vi "Main.vi"() -> ()   [LabVIEW 2016]
uses:
  Data Highway TD.ctl
  Queue Attributes TD.ctl
  Que Enum td.ctl
panel:
  in  "Log":bool
  in  "PP_value":dbl
  in  "PP_HOME":bool
  in  "PP_STOP":bool
  in  "PP_START":bool
  in  "Connect":bool
  in  "Exit":bool
  # "Pitchpack"
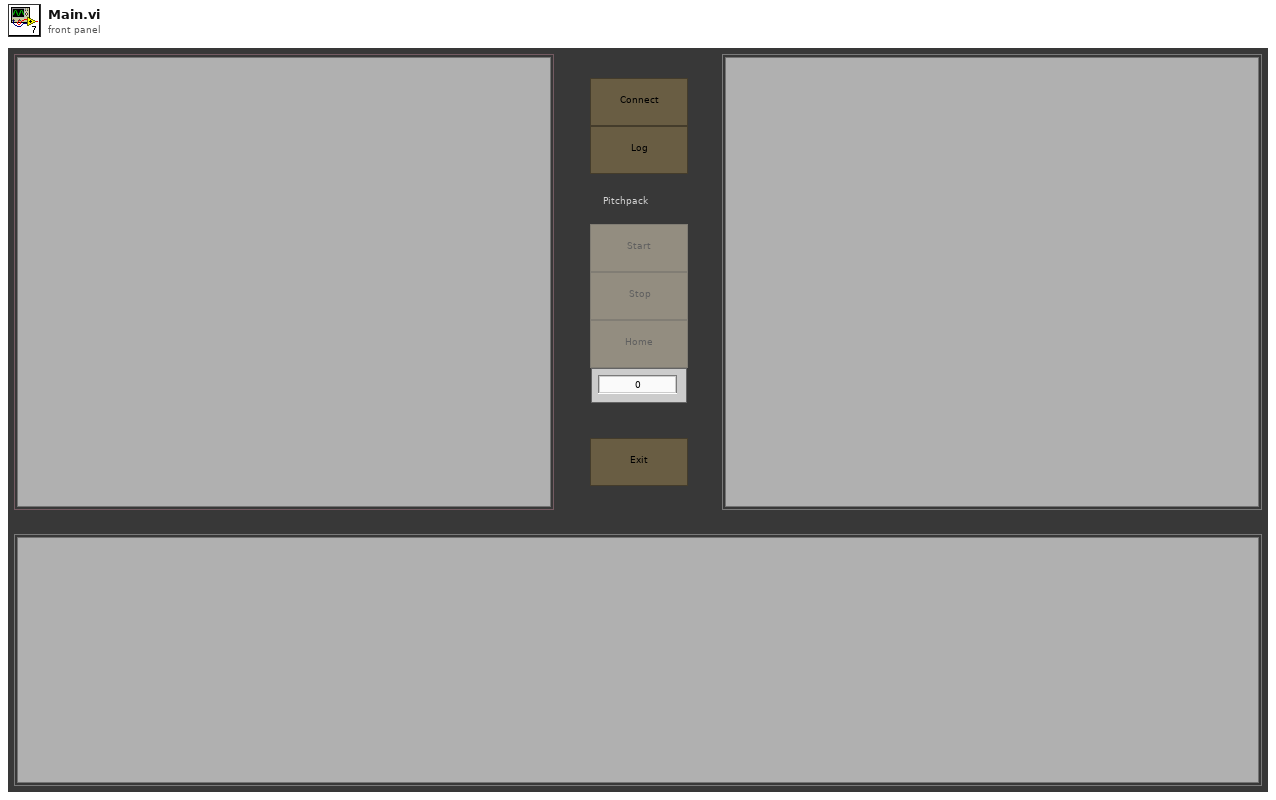
[diagram p1: front panel]
types:
  T1 = typedef "Data Highway TD.ctl" = cluster{"PP_value":dbl, "String":string, "Boolean":bool}
  T2 = typedef "Que Cluster TD.ctl" = cluster{"Main":refnum<queue>, "ZMQ_SUB":refnum<queue>, "External":refnum<queue>, "Vibration":refnum<queue>, "ZMQ_REQ":refnum<queue>}
  T3 = typedef "Queue Attributes TD.ctl" = cluster{"Que States":T4, "String":string, "Boolean":bool, "Double":dbl, "U16":u16}
  T4 = typedef "Que enum td.ctl" = enum16{"Stop", "Start", "Update D_HW", "Initialize", "Exit", "Read", "Write", "Plot", "Log", "Stop Log", "Start Log", "Wait"}
  T5 = typedef "Que Atributes TD.ctl" = cluster{"Que States":T4, "String":string, "Boolean":bool, "Double":dbl, "U16":u16}
  T6 = enum8{"Enabled", "Disabled", "Disabled and Grayed Out"}
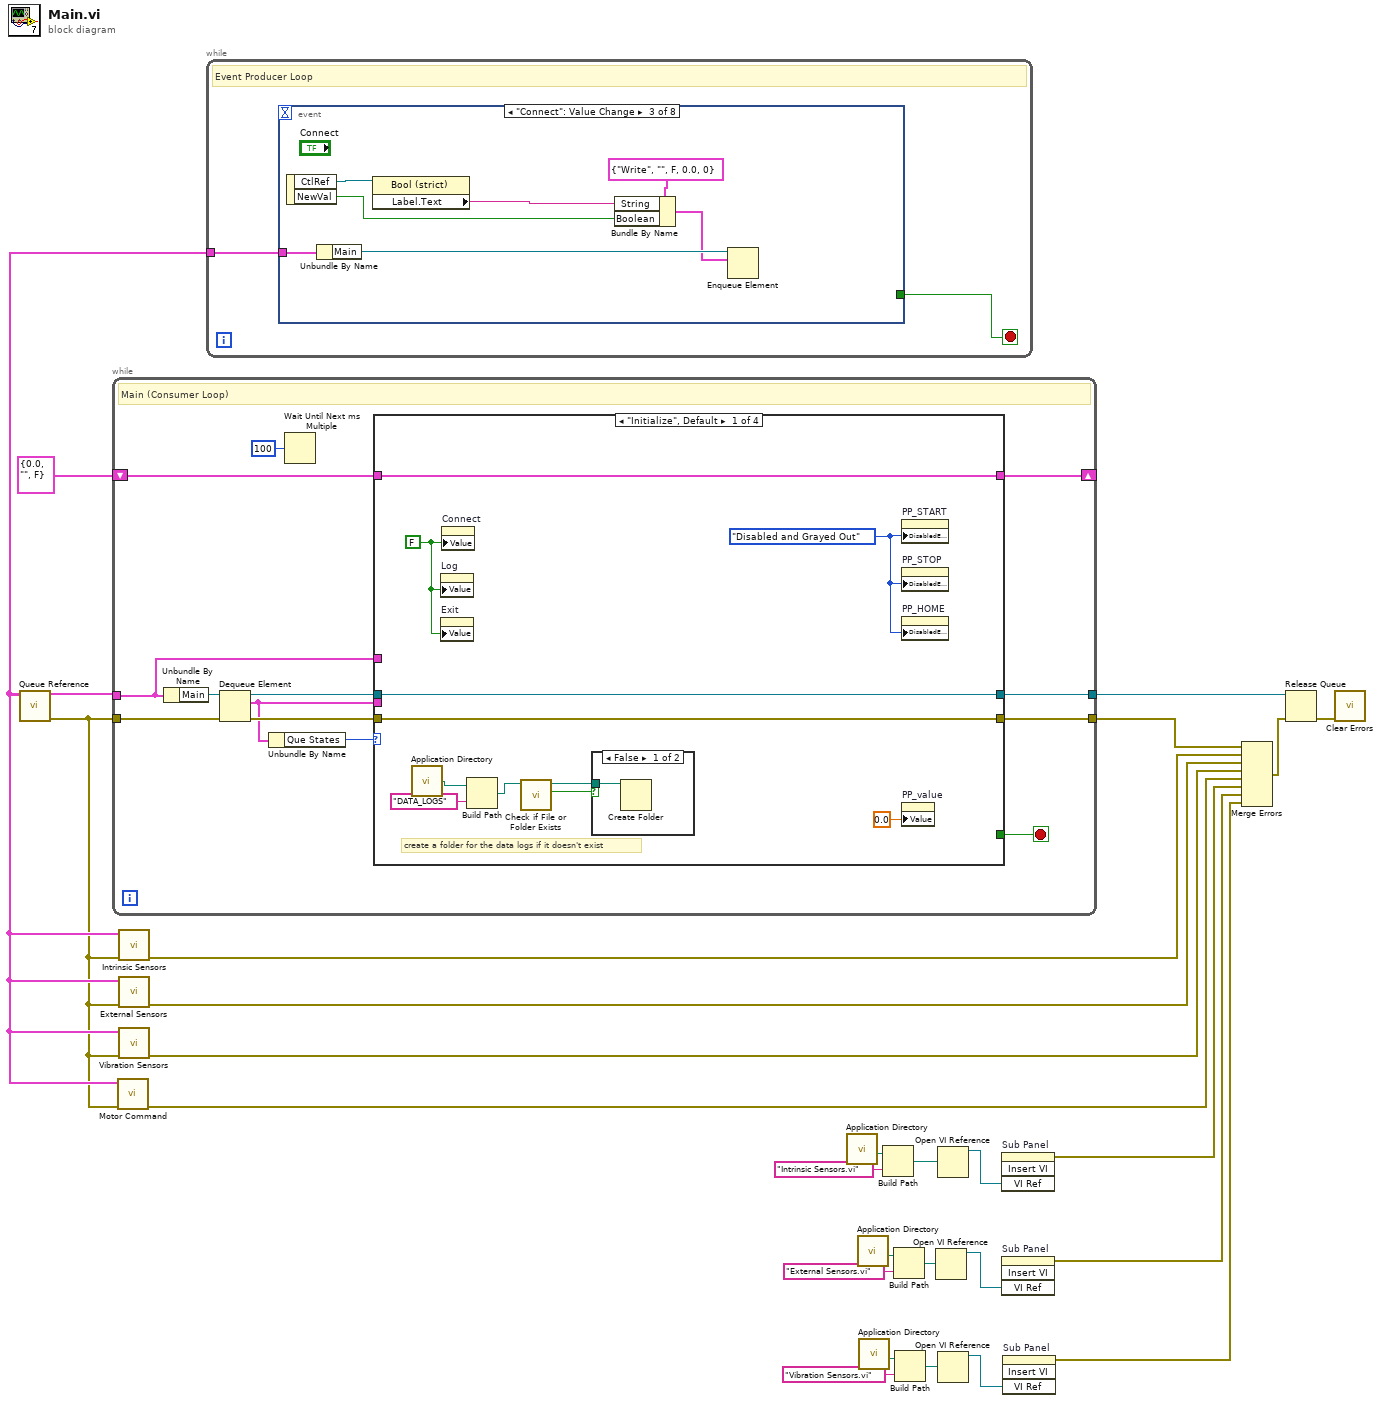
[diagram p0: block diagram]
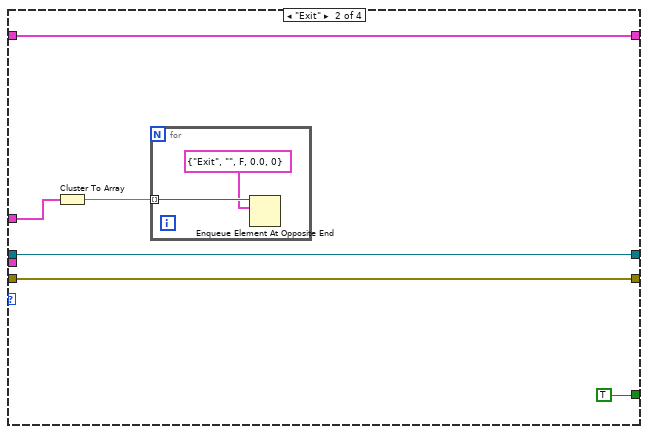
[diagram p3: hidden frame]
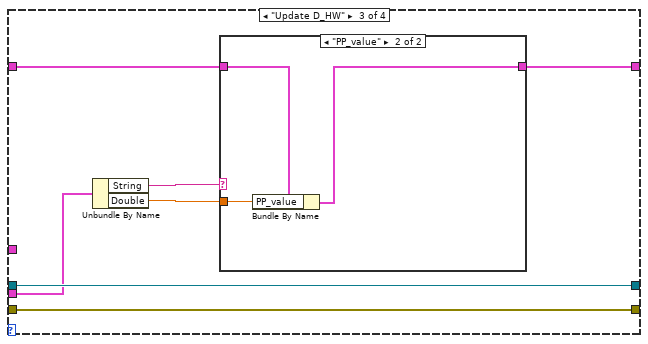
[diagram p4: hidden frame]
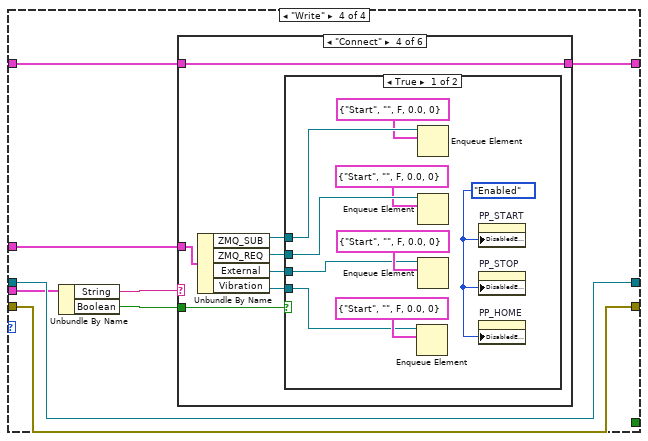
[diagram p6: hidden frame]
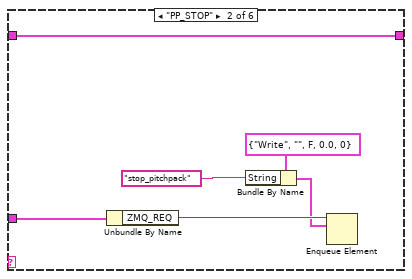
[diagram p8: hidden frame]
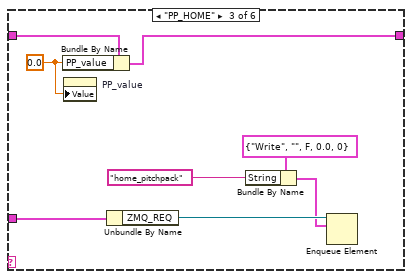
[diagram p9: hidden frame]
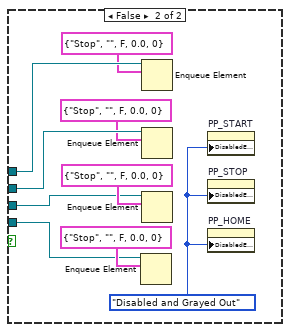
[diagram p10: hidden frame]
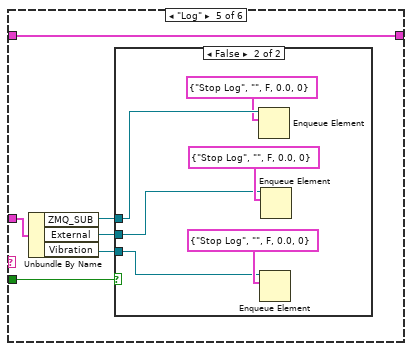
[diagram p11: hidden frame]
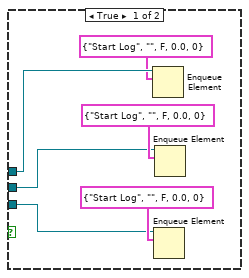
[diagram p12: hidden frame]
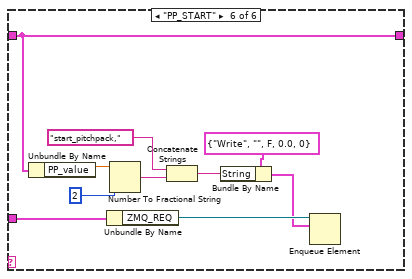
[diagram p13: hidden frame]
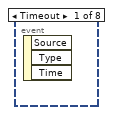
[diagram p14: hidden frame]
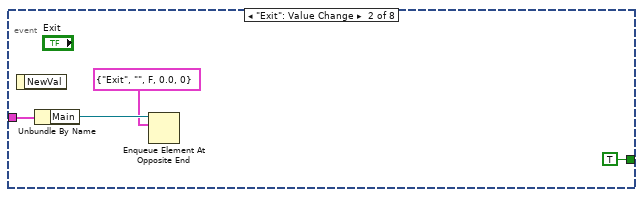
[diagram p15: hidden frame]
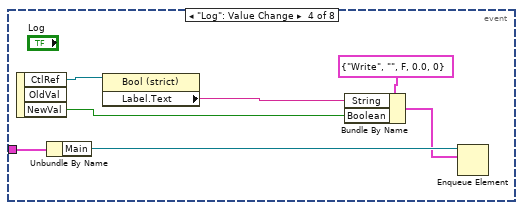
[diagram p16: hidden frame]
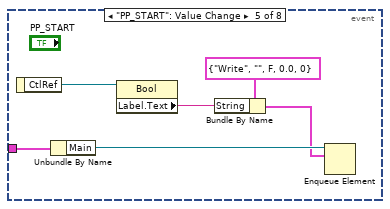
[diagram p17: hidden frame]
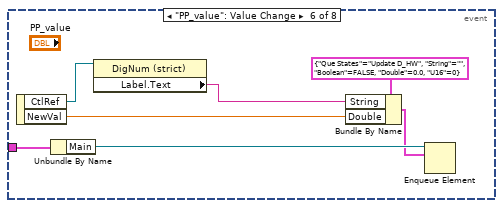
[diagram p18: hidden frame]
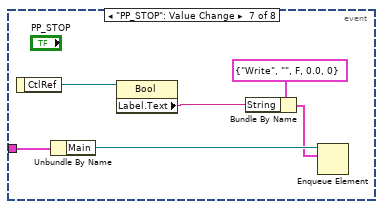
[diagram p19: hidden frame]
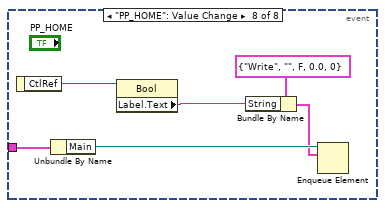
[diagram p20: hidden frame]
diagram:
  n1 = call "Queue Reference.vi"() -> ("error out"=w2:errorcluster, "output cluster"=w3:T2)  [unwired: 10 in]
  n2 = while {
    tunnel: w2 -> [w38]
    tunnel: w3 -> [w32]
    tunnel: [w35] -> w26
    tunnel: [w34] -> w24
    shift-right: [w30] -> _
    shift-left: T1 {"PP_value"=0.0, "String"="", "Boolean"=FALSE} ("Data Hyway") -> [w31]
    stop <- w28 stop-if-true
    # "Main (Consumer Loop)"
    n3 = Unbundle By Name(w32) -> ("Main"=w39:refnum<queue>)
    n4 = Dequeue Element(queue=w39, error in (no error)=w38) -> (queue out=w37:refnum<queue>, element=w27:T5, error out=w36:errorcluster)  [unwired: 1 in, 1 out]
    n5 = Unbundle By Name(w27) -> ("Que States"=w33:T4)
    n6 = Wait Until Next ms Multiple(millisecond multiple=u32 100) -> ()  [unwired: 1 out]
    n7 = case shown="\"Initialize\", Default" w33 {
      tunnel: w37 -> [w50 w57 w66 w77]
      tunnel: w36 -> [w49 w56 w63 w72]
      tunnel: [w50 w57 w66 w77] -> w35
      tunnel: [w49 w56 w63 w72] -> w34
      tunnel: w32 -> [_ w54 _ w78]
      tunnel: w31 -> [w48 w55 w65 w76]
      tunnel: [w48 w55 w64 w75] -> w30
      tunnel: [_ TRUE _ _] -> w28
      tunnel: w27 -> [_ _ w62 w74]
      frame "Initialize", Default {
        w45 = FALSE ("Connect")
        w47 = T6."Disabled and Grayed Out" ("Disabled")
        # "create a folder for the data logs if it doesn't exist"
        n8 = call <vilib>:"Application Directory.vi"() -> ("Application Directory"=w42:path)
        n9 = property on="Log" class="Bool (strict)"("Value"=w45) -> ()  [unwired: 2 in, 2 out]
        n10 = property on="Exit" class="Bool (strict)"("Value"=w45) -> ()  [unwired: 2 in, 2 out]
        n11 = property on="Connect" class="Bool (strict)"("Value"=w45) -> ()  [unwired: 2 in, 2 out]
        n12 = Build Path(base path=w42, name or relative path="DATA_LOGS") -> (appended path=w44:path)
        n13 = call <vilib>:"Check if File or Folder Exists.vi"("path"=w44) -> ("file or folder exists?"=w41:bool, "dup path"=w40:path)  [unwired: 8 in, 1 out]
        n14 = case shown="False" w41 {
          tunnel: w40 -> [w51 _]
          frame False {
            n15 = Create Folder(path (use dialog)=w51) -> ()  [unwired: 2 in, 3 out]
          }
          frame True {
          }
        }
        n16 = property on="PP_START" class="Bool"("DisabledEnum"=w47) -> ()  [unwired: 2 in, 2 out]
        n17 = property on="PP_STOP" class="Bool"("DisabledEnum"=w47) -> ()  [unwired: 2 in, 2 out]
        n18 = property on="PP_HOME" class="Bool"("DisabledEnum"=w47) -> ()  [unwired: 2 in, 2 out]
        n19 = property on="PP_value" class="DigNum (strict)"("Value"=0.0 ("PP_value")) -> ()  [unwired: 2 in, 2 out]
      }
      frame "Exit" {
        n20 = Cluster To Array(cluster=w54) -> (array=w53:refnum<queue>[])
        n21 = for {
          tunnel: w53 -> [w59] mode=indexing
          n22 = Enqueue Element At Opposite End(queue=w59, element=T3 {"Que States"=enum."Exit", "String"="", "Boolean"=FALSE, "Double"=0.0, "U16"=0}) -> ()  [unwired: 2 in, 3 out]
        }
      }
      frame "Update D_HW" {
        n23 = Unbundle By Name(w62) -> ("String"=w61:string, "Double"=w60:dbl)
        n24 = case shown="\"PP_value\"" w61 {
          tunnel: w65 -> [w67 w70]
          tunnel: [w67 w69] -> w64
          tunnel: w60 -> [_ w68]
          frame "False", Default {
          }
          frame "PP_value" {
            n25 = Bundle By Name(cluster=w70, "PP_value"=w68) -> (w69:T1)
          }
        }
      }
      frame "Write" {
        n26 = Unbundle By Name(w74) -> ("String"=w73:string, "Boolean"=w71:bool)
        n27 = case shown="\"Connect\"" w73 {
          tunnel: w78 -> [_ w85 w93 w99 w123 w146]
          tunnel: w76 -> [w79 w82 w90 w100 w124 w141]
          tunnel: [w79 w82 w89 w100 w124 w141] -> w75
          tunnel: w71 -> [_ _ _ w96 w121 _]
          frame "False", Default {
          }
          frame "PP_STOP" {
            n28 = Unbundle By Name(w85) -> ("ZMQ_REQ"=w84:refnum<queue>)
            n29 = Bundle By Name(cluster=T3 {"Que States"=enum."Write", "String"="", "Boolean"=FALSE, "Double"=0.0, "U16"=0} ("element"), "String"="stop_pitchpack") -> (w80:T3)
            n30 = Enqueue Element(queue=w84, element=w80) -> ()  [unwired: 2 in, 3 out]
          }
          frame "PP_HOME" {
            w86 = 0.0 ("PP_value")
            n31 = Bundle By Name(cluster=w90, "PP_value"=w86) -> (w89:T1)
            n32 = property on="PP_value" class="DigNum (strict)"("Value"=w86) -> ()  [unwired: 2 in, 2 out]
            n33 = Unbundle By Name(w93) -> ("ZMQ_REQ"=w92:refnum<queue>)
            n34 = Bundle By Name(cluster=T3 {"Que States"=enum."Write", "String"="", "Boolean"=FALSE, "Double"=0.0, "U16"=0} ("element"), "String"="home_pitchpack") -> (w87:T3)
            n35 = Enqueue Element(queue=w92, element=w87) -> ()  [unwired: 2 in, 3 out]
          }
          frame "Connect" {
            n36 = Unbundle By Name(w99) -> ("ZMQ_SUB"=w98:refnum<queue>, "ZMQ_REQ"=w97:refnum<queue>, "External"=w95:refnum<queue>, "Vibration"=w94:refnum<queue>)
            n37 = case shown="True" w96 {
              tunnel: w98 -> [w109 w118]
              tunnel: w97 -> [w108 w117]
              tunnel: w95 -> [w103 w112]
              tunnel: w94 -> [w101 w110]
              frame True {
                w107 = T6."Enabled" ("Disabled")
                n38 = Enqueue Element(queue=w101, element=T3 {"Que States"=enum."Start", "String"="", "Boolean"=FALSE, "Double"=0.0, "U16"=0}) -> ()  [unwired: 2 in, 3 out]
                n39 = Enqueue Element(queue=w109, element=T3 {"Que States"=enum."Start", "String"="", "Boolean"=FALSE, "Double"=0.0, "U16"=0}) -> ()  [unwired: 2 in, 3 out]
                n40 = Enqueue Element(queue=w108, element=T3 {"Que States"=enum."Start", "String"="", "Boolean"=FALSE, "Double"=0.0, "U16"=0}) -> ()  [unwired: 2 in, 3 out]
                n41 = Enqueue Element(queue=w103, element=T3 {"Que States"=enum."Start", "String"="", "Boolean"=FALSE, "Double"=0.0, "U16"=0}) -> ()  [unwired: 2 in, 3 out]
                n42 = property on="PP_START" class="Bool"("DisabledEnum"=w107) -> ()  [unwired: 2 in, 2 out]
                n43 = property on="PP_STOP" class="Bool"("DisabledEnum"=w107) -> ()  [unwired: 2 in, 2 out]
                n44 = property on="PP_HOME" class="Bool"("DisabledEnum"=w107) -> ()  [unwired: 2 in, 2 out]
              }
              frame False {
                w116 = T6."Disabled and Grayed Out" ("Disabled")
                n45 = Enqueue Element(queue=w110, element=T3 {"Que States"=enum."Stop", "String"="", "Boolean"=FALSE, "Double"=0.0, "U16"=0}) -> ()  [unwired: 2 in, 3 out]
                n46 = Enqueue Element(queue=w118, element=T3 {"Que States"=enum."Stop", "String"="", "Boolean"=FALSE, "Double"=0.0, "U16"=0}) -> ()  [unwired: 2 in, 3 out]
                n47 = Enqueue Element(queue=w117, element=T3 {"Que States"=enum."Stop", "String"="", "Boolean"=FALSE, "Double"=0.0, "U16"=0}) -> ()  [unwired: 2 in, 3 out]
                n48 = Enqueue Element(queue=w112, element=T3 {"Que States"=enum."Stop", "String"="", "Boolean"=FALSE, "Double"=0.0, "U16"=0}) -> ()  [unwired: 2 in, 3 out]
                n49 = property on="PP_START" class="Bool"("DisabledEnum"=w116) -> ()  [unwired: 2 in, 2 out]
                n50 = property on="PP_STOP" class="Bool"("DisabledEnum"=w116) -> ()  [unwired: 2 in, 2 out]
                n51 = property on="PP_HOME" class="Bool"("DisabledEnum"=w116) -> ()  [unwired: 2 in, 2 out]
              }
            }
          }
          frame "Log" {
            n52 = Unbundle By Name(w123) -> ("ZMQ_SUB"=w122:refnum<queue>, "External"=w120:refnum<queue>, "Vibration"=w119:refnum<queue>)
            n53 = case shown="False" w121 {
              tunnel: w122 -> [w130 w136]
              tunnel: w120 -> [w127 w133]
              tunnel: w119 -> [w125 w131]
              frame True {
                n54 = Enqueue Element(queue=w130, element=T3 {"Que States"=enum."Start Log", "String"="", "Boolean"=FALSE, "Double"=0.0, "U16"=0}) -> ()  [unwired: 2 in, 3 out]
                n55 = Enqueue Element(queue=w125, element=T3 {"Que States"=enum."Start Log", "String"="", "Boolean"=FALSE, "Double"=0.0, "U16"=0}) -> ()  [unwired: 2 in, 3 out]
                n56 = Enqueue Element(queue=w127, element=T3 {"Que States"=enum."Start Log", "String"="", "Boolean"=FALSE, "Double"=0.0, "U16"=0}) -> ()  [unwired: 2 in, 3 out]
              }
              frame False {
                n57 = Enqueue Element(queue=w136, element=T3 {"Que States"=enum."Stop Log", "String"="", "Boolean"=FALSE, "Double"=0.0, "U16"=0}) -> ()  [unwired: 2 in, 3 out]
                n58 = Enqueue Element(queue=w131, element=T3 {"Que States"=enum."Stop Log", "String"="", "Boolean"=FALSE, "Double"=0.0, "U16"=0}) -> ()  [unwired: 2 in, 3 out]
                n59 = Enqueue Element(queue=w133, element=T3 {"Que States"=enum."Stop Log", "String"="", "Boolean"=FALSE, "Double"=0.0, "U16"=0}) -> ()  [unwired: 2 in, 3 out]
              }
            }
          }
          frame "PP_START" {
            n60 = Unbundle By Name(w141) -> ("PP_value"=w144:dbl)
            n61 = Unbundle By Name(w146) -> ("ZMQ_REQ"=w145:refnum<queue>)
            n62 = Number To Fractional String(number=w144, precision (6)=i16 2) -> (F-format string=w142:string)  [unwired: 2 in]
            n63 = Concatenate Strings("start_pitchpack,", w142) -> (w139:string)
            n64 = Bundle By Name(cluster=T3 {"Que States"=enum."Write", "String"="", "Boolean"=FALSE, "Double"=0.0, "U16"=0} ("element"), "String"=w139) -> (w138:T3)
            n65 = Enqueue Element(queue=w145, element=w138) -> ()  [unwired: 2 in, 3 out]
          }
        }
      }
    }
  }
  n66 = call "Motor Command.vi"("error in (no error)"=w2, "output cluster"=w3) -> ("error out"=w1:errorcluster)  [unwired: 9 in]
  n67 = call "Intrinsic Sensors.vi"("error in (no error)"=w2, "output cluster"=w3) -> ("error out"=w19:errorcluster)  [unwired: 9 in]
  n68 = call "External Sensors.vi"("error in (no error)"=w2, "output cluster"=w3) -> ("error out"=w5:errorcluster)  [unwired: 9 in]
  n69 = call "Vibration Sensors.vi"("error in (no error)"=w2, "output cluster"=w3) -> ("error out"=w4:errorcluster)  [unwired: 9 in]
  n70 = while {
    tunnel: w3 -> [w148]
    stop <- w147 stop-if-true
    # "Event Producer Loop"
    n71 = event shown="[2] \"Connect\": Value Change" {
      selector: _ -> [_ _ _ _ _ _ _ _]
      dyn-events: _ -> [_ _ _ _ _ _ _ _]
      timeout: _ -> [_ _ _ _ _ _ _ _]
      tunnel: w148 -> [_ w152 w159 w166 w172 w179 w185 w191]
      tunnel: [_ TRUE ("User Event") _ _ _ _ _ _] -> w147
      event Timeout {
        n72 = event-data() -> ()  [unwired: 1 in, 3 out]
      }
      event "Exit": Value Change {
        n73 = event-data() -> ()  [unwired: 1 in, 1 out]
        n74 = Unbundle By Name(w152) -> ("Main"=w151:refnum<queue>)
        n75 = Enqueue Element At Opposite End(queue=w151, element=T3 {"Que States"=enum."Exit", "String"="", "Boolean"=FALSE, "Double"=0.0, "U16"=0}) -> ()  [unwired: 2 in, 3 out]
      }
      event "Connect": Value Change {
        n76 = event-data() -> ("CtlRef"=w157:refnum<vi>, "NewVal"=w154:bool)  [unwired: 1 in]
        n77 = Unbundle By Name(w159) -> ("Main"=w158:refnum<queue>)
        n78 = property class="Bool (strict)"(reference=w157) -> ("Label.Text"=w155:string)  [unwired: 1 in, 2 out]
        n79 = Bundle By Name(cluster=T3 {"Que States"=enum."Write", "String"="", "Boolean"=FALSE, "Double"=0.0, "U16"=0} ("element"), "String"=w155, "Boolean"=w154) -> (w153:T3)
        n80 = Enqueue Element(queue=w158, element=w153) -> ()  [unwired: 2 in, 3 out]
      }
      event "Log": Value Change {
        n81 = event-data() -> ("CtlRef"=w164:refnum<vi>, "NewVal"=w160:bool)  [unwired: 1 in, 1 out]
        n82 = Unbundle By Name(w166) -> ("Main"=w165:refnum<queue>)
        n83 = property class="Bool (strict)"(reference=w164) -> ("Label.Text"=w162:string)  [unwired: 1 in, 2 out]
        n84 = Bundle By Name(cluster=T3 {"Que States"=enum."Write", "String"="", "Boolean"=FALSE, "Double"=0.0, "U16"=0} ("element"), "String"=w162, "Boolean"=w160) -> (w161:T3)
        n85 = Enqueue Element(queue=w165, element=w161) -> ()  [unwired: 2 in, 3 out]
      }
      event "PP_START": Value Change {
        n86 = event-data() -> ("CtlRef"=w170:refnum<vi>)  [unwired: 1 in]
        n87 = Unbundle By Name(w172) -> ("Main"=w171:refnum<queue>)
        n88 = property class="Bool"(reference=w170) -> ("Label.Text"=w169:string)  [unwired: 1 in, 2 out]
        n89 = Bundle By Name(cluster=T3 {"Que States"=enum."Write", "String"="", "Boolean"=FALSE, "Double"=0.0, "U16"=0} ("element"), "String"=w169) -> (w167:T3)
        n90 = Enqueue Element(queue=w171, element=w167) -> ()  [unwired: 2 in, 3 out]
      }
      event "PP_value": Value Change {
        n91 = event-data() -> ("CtlRef"=w177:refnum<vi>, "NewVal"=w174:dbl)  [unwired: 1 in]
        n92 = Unbundle By Name(w179) -> ("Main"=w178:refnum<queue>)
        n93 = property class="DigNum (strict)"(reference=w177) -> ("Label.Text"=w175:string)  [unwired: 1 in, 2 out]
        n94 = Bundle By Name(cluster=T3 {"Que States"=enum."Update D_HW", "String"="", "Boolean"=FALSE, "Double"=0.0, "U16"=0} ("element"), "String"=w175, "Double"=w174) -> (w173:T3)
        n95 = Enqueue Element(queue=w178, element=w173) -> ()  [unwired: 2 in, 3 out]
      }
      event "PP_STOP": Value Change {
        n96 = event-data() -> ("CtlRef"=w183:refnum<vi>)  [unwired: 1 in]
        n97 = Unbundle By Name(w185) -> ("Main"=w184:refnum<queue>)
        n98 = property class="Bool"(reference=w183) -> ("Label.Text"=w181:string)  [unwired: 1 in, 2 out]
        n99 = Bundle By Name(cluster=T3 {"Que States"=enum."Write", "String"="", "Boolean"=FALSE, "Double"=0.0, "U16"=0} ("element"), "String"=w181) -> (w180:T3)
        n100 = Enqueue Element(queue=w184, element=w180) -> ()  [unwired: 2 in, 3 out]
      }
      event "PP_HOME": Value Change {
        n101 = event-data() -> ("CtlRef"=w189:refnum<vi>)  [unwired: 1 in]
        n102 = Unbundle By Name(w191) -> ("Main"=w190:refnum<queue>)
        n103 = property class="Bool"(reference=w189) -> ("Label.Text"=w187:string)  [unwired: 1 in, 2 out]
        n104 = Bundle By Name(cluster=T3 {"Que States"=enum."Write", "String"="", "Boolean"=FALSE, "Double"=0.0, "U16"=0} ("element"), "String"=w187) -> (w186:T3)
        n105 = Enqueue Element(queue=w190, element=w186) -> ()  [unwired: 2 in, 3 out]
      }
    }
  }
  n106 = call <vilib>:"Application Directory.vi"() -> ("Application Directory"=w14:path)
  n107 = call <vilib>:"Application Directory.vi"() -> ("Application Directory"=w10:path)
  n108 = call <vilib>:"Application Directory.vi"() -> ("Application Directory"=w8:path)
  n109 = Build Path(base path=w14, name or relative path="Intrinsic Sensors.vi") -> (appended path=w12:path)
  n110 = Build Path(base path=w10, name or relative path="External Sensors.vi") -> (appended path=w9:path)
  n111 = Build Path(base path=w8, name or relative path="Vibration Sensors.vi") -> (appended path=w6:path)
  n112 = Open VI Reference(vi path=w9) -> (vi reference=w20:refnum<vi>)  [unwired: 5 in, 1 out]
  n113 = Open VI Reference(vi path=w12) -> (vi reference=w22:refnum<vi>)  [unwired: 5 in, 1 out]
  n114 = Open VI Reference(vi path=w6) -> (vi reference=w18:refnum<vi>)  [unwired: 5 in, 1 out]
  n115 = invoke on="Sub Panel" class="SubPnl" method="Insert VI"("VI Ref"=w22) -> (error out=w15:errorcluster)  [unwired: 3 in, 3 out]
  n116 = invoke on="Sub Panel" class="SubPnl" method="Insert VI"("VI Ref"=w20) -> (error out=w16:errorcluster)  [unwired: 3 in, 3 out]
  n117 = invoke on="Sub Panel" class="SubPnl" method="Insert VI"("VI Ref"=w18) -> (error out=w17:errorcluster)  [unwired: 3 in, 3 out]
  n118 = Merge Errors(w24, w19, w5, w4, w1, w15, w16, w17) -> (w23:errorcluster)
  n119 = Release Queue(queue=w26, error in (no error)=w23) -> (error out=w21:errorcluster)  [unwired: 1 in, 2 out]
  n120 = call <vilib>:"Clear Errors.vi"("error in (no error)"=w21) -> ()  [unwired: 5 in, 2 out]
